vi "Right way.vi"() -> ()   [LabVIEW 2016]
panel:
  out "before substring 3":string
  out "before substring 2":string
  out "before substring":string
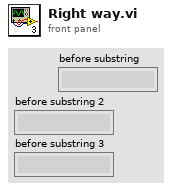
[diagram p1: front panel]
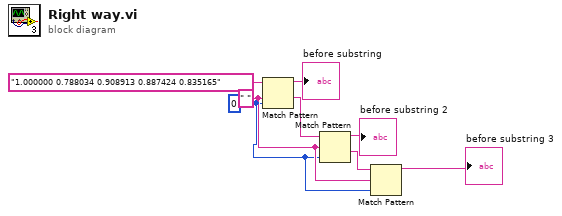
[diagram p0: block diagram]
diagram:
  w3 = 0 ("offset (0)")
  w4 = " " ("regular expression")
  n1 = Match Pattern(string="1.000000 0.788034 0.908913 0.887424 0.835165", regular expression=w4, offset (0)=w3) -> (before substring=→"before substring":string, after substring=w6:string)  [unwired: 2 out]
  n2 = Match Pattern(string=w6, regular expression=w4, offset (0)=w3) -> (before substring=→"before substring 2":string, after substring=w5:string)  [unwired: 2 out]
  n3 = Match Pattern(string=w5, regular expression=w4, offset (0)=w3) -> (before substring=→"before substring 3":string)  [unwired: 3 out]
